vi "setFilter.vi"(8 "error in (no error)":errorcluster, 10 "Filter Type":T1, 11 "ZTAAC in":refnum<class "ZTAAC.lvclass">) -> (0 "error out":errorcluster, 3 "ZTAAC out":refnum<class "ZTAAC.lvclass">)   [LabVIEW 2016, in "OfcFunc.lvlib" / "ZTAAC.lvclass"]
doc: "Set the active filter type."
uses:
  ZTAAC.lvclass
  StrictDef/FilterType.ctl
  ZTAAC.lvclass/ZTAAC.ctl
  OfcFunc.lvlib
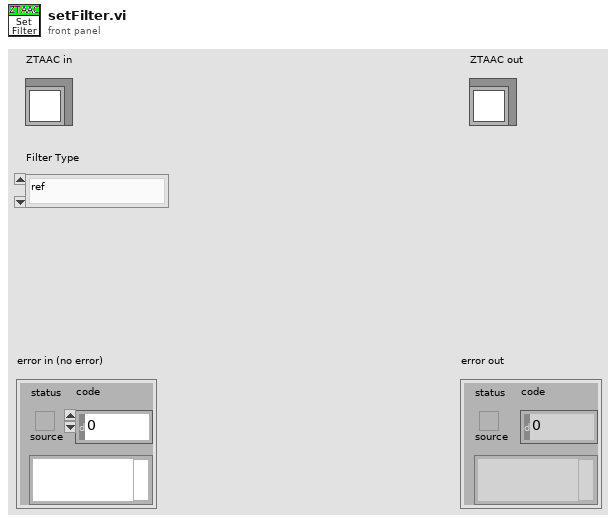
[diagram p1: front panel]
types:
  T1 = typedef "OfcFunc.lvlib/FilterType.ctl" = enum16{"ref", "u", "g", "r", "i", "z", "y"}
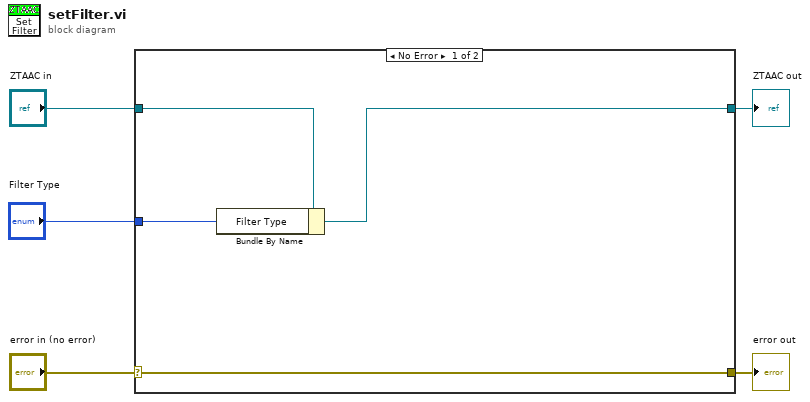
[diagram p0: block diagram]
diagram:
  n1 = case shown="No Error" "error in (no error)" {
    selector: "error in (no error)" -> [w9 w11]
    tunnel: [w9 w11] -> w4
    tunnel: [w6 w10] -> w2
    tunnel: "ZTAAC in" -> [w8 w10]
    tunnel: "Filter Type" -> [w7 _]
    frame No Error {
      n2 = Bundle By Name(cluster=w8, "Filter Type"=w7) -> (w6:refnum<class "ZTAAC.lvclass">)
    }
    frame Error {
    }
  }
  "error out" <- w4
  "ZTAAC out" <- w2
